vi "SQL_EDITOR_prepare_DELETE_statement.vi"(7 "nmb_of_top_rows (all)":i32, 8 "error_in":errorcluster, 10 "selected_record":i32, 11 "SQL_EDIT_records":string[][](array[string])) -> (0 "error_out":errorcluster, 3 "DELETE_statement":string)   [LabVIEW 2019]
uses:
  FGV/SQL_EDITOR_records_display/FGV_SQL_EDITOR_records_display.ctl
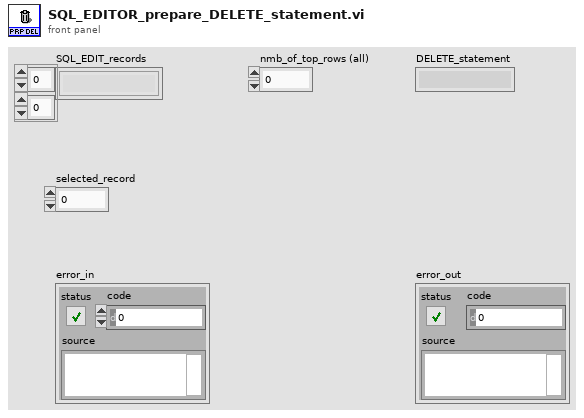
[diagram p1: front panel]
types:
  T1 = typedef "FGV_SQL_EDITOR_records_display.ctl" = enum16{"initialize", "set_table_name", "set_column_name", "set_value_to_select", "set_order_by", "set_asc_desc", "set_headers", "set_records", "get_table_name", "get_column_name", "get_value_to_select", "get_headers", "get_all_info", "record_added?", "record_inserted?", "record_edited?", "record_updated?", "record_deleted?", "discard_changes"}
  T2 = typedef "SQL_EDITOR_all_info.ctl" = cluster{"table":string, "column":string, "value_to_select":string, "order_by":string, "asc_desc":string, "headers":string[], "uneditable_columns":string[], "uneditable_columns":i32[], "editable_columns":i32[], "values_in_database":string[][], "size":cluster{"columns":i32, "SQL_rows":i32, "disp_rows":i32}, "SQL_record_states":T3[]}
  T3 = typedef "SQL_record_states.ctl" = enum16{"Equal", "Added", "Edited", "Deleted"}
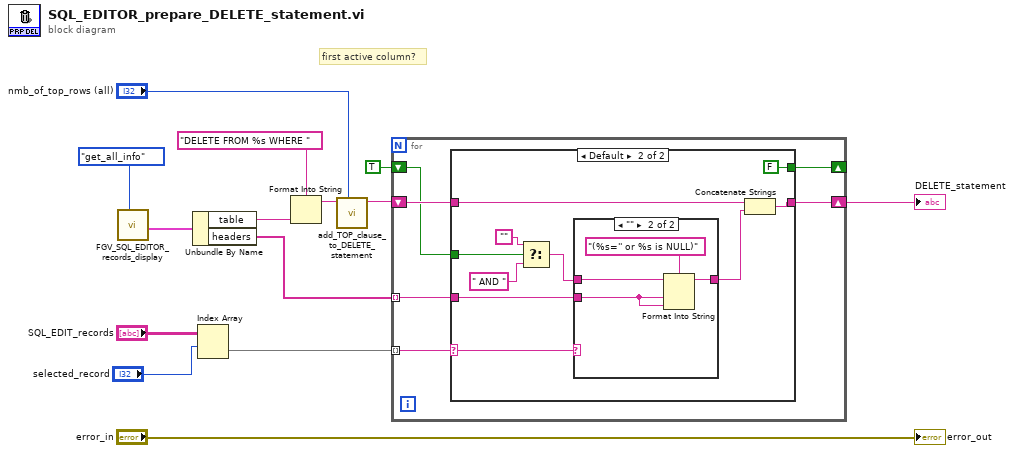
[diagram p0: block diagram]
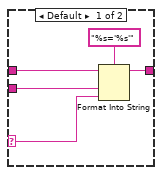
[diagram p3: hidden frame]
diagram:
  # "first active column?"
  n1 = call "FGV_SQL_EDITOR_records_display.vi"("options"=FGV_SQL_EDITOR_records_display."get_all_info") -> ("all_info"=w5:T2)  [unwired: 7 in, 3 out]
  n2 = Unbundle By Name(w5) -> ("table"=w8:string, "headers"=w9:string[])
  n3 = Index Array(array="SQL_EDIT_records", index (row)="selected_record") -> (element=w2:string[])  [unwired: 1 in]
  n4 = Format Into String(format string="DELETE FROM %s WHERE ", w8) -> (resulting string=w11:string)  [unwired: 2 in, 1 out]
  n5 = call "add_TOP_clause_to_DELETE_statement.vi"("nmb_of_top_rows (all)"="nmb_of_top_rows (all)", "DELETE_statement_in"=w11) -> ("DELETE_statement_out"=w13:string)  [unwired: 8 in, 1 out]
  n6 = for {
    tunnel: w2 -> [w18] mode=indexing
    tunnel: w9 -> [w19] mode=indexing
    shift-right: [w17] -> w14
    shift-left: w13 -> [w20]
    shift-right: [w15] -> _
    shift-left: TRUE -> [w16]
    n7 = case shown="Default" w18 {
      selector: w18 -> [_ w27]
      tunnel: w20 -> [w22 w30]
      tunnel: w19 -> [_ w28]
      tunnel: [w22 w25] -> w17
      tunnel: w16 -> [w21 w24]
      tunnel: [w21 FALSE] -> w15
      frame "" {
      }
      frame Default {
        n8 = Select(t="", s=w24, f=" AND ") -> (s? t:f=w29:string)
        n9 = case shown="\"\"" w27 {
          selector: w27 -> [w34 _]
          tunnel: w29 -> [w36 w40]
          tunnel: w28 -> [w35 w38]
          tunnel: [w33 w39] -> w26
          frame Default {
            n10 = Format Into String(format string="%s='%s'", initial string=w36, w35, w34) -> (resulting string=w33:string)  [unwired: 1 in, 1 out]
          }
          frame "" {
            n11 = Format Into String(format string="(%s='' or %s is NULL)", initial string=w40, w38, w38) -> (resulting string=w39:string)  [unwired: 1 in, 1 out]
          }
        }
        n12 = Concatenate Strings(w30, w26) -> (w25:string)
      }
    }
  }
  "DELETE_statement" <- w14
  "error_out" <- "error_in"
